vi "Test - Thermal Chamber Controller_DQMH - Update Ramp Rate 1-teardown.vi"(7 "test case ID":string, 8 "error in (no error)":errorcluster, 10 "Temperature Ramp Rate":dbl format="%#_13g", 11 "no error":bool) -> (0 "error out":errorcluster, 3 "result":bool)   [LabVIEW 2015]
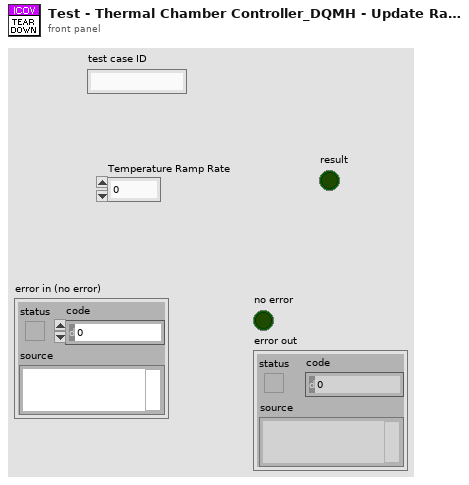
[diagram p1: front panel]
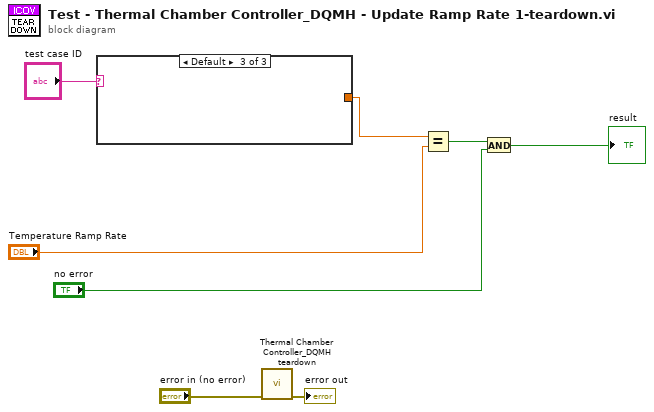
[diagram p0: block diagram]
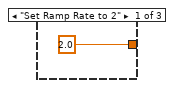
[diagram p2: hidden frame]
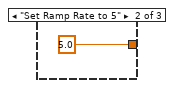
[diagram p3: hidden frame]
diagram:
  n1 = case shown="Default" "test case ID" {
    tunnel: [2.0 ("Temperature Ramp Rate 2") 5.0 ("Temperature Ramp Rate 2") _] -> w1
    frame "Set Ramp Rate to 2" {
    }
    frame "Set Ramp Rate to 5" {
    }
    frame Default {
    }
  }
  n2 = call "Thermal Chamber Controller_DQMH teardown.vi"("error in (no error)"="error in (no error)") -> ("error out"=→"error out":errorcluster)  [unwired: 10 in]
  n3 = Equal?(x=w1, y="Temperature Ramp Rate") -> (x = y?=w7:bool)
  n4 = And(x=w7, y="no error") -> (x .and. y?=→"result":bool)
